vi "TalonSRXSetStatusRates.vi"(9 "Talon SRX Set Status Rates":T1={"General (ms)"=10, "Feedback 0 (ms)"=5, "Ain, Temp, Vbat (ms)"=255, "Misc (ms)"=255, "Comm Status (ms)"=255, "Mot Prof Buffer (ms)"=255, "Motion Magic (ms)"=255, "Firmware API Status (ms)"=255, "PIDF 1 (ms)"=255, "PIDF 0 (ms)"=255, "Feedback 1 (ms)"=255}, 11 "Talon SRX DevRef In":T2={"DeviceStatus"={"status"=FALSE, "code"=0, "source"=""}, "Type"=enum."PWM", "PWM"={"PWM Channel"=enum."PWM 1", "DeadBand"={"Name"="", "maxPositivePwm"=0, "minPositivePwm"=0, "centerPwm"=0, "maxNegativePwm"=0, "minNegativePwm"=0, "angularRange"=0}}, "CAN"={"Device Number"=0, "SetOutput VI Ref"=variant(enum8{"Percent VBus", "Current", "Speed", "Position", "Voltage"} enum."Percent VBus"), "GetOutput VI Ref"=variant(refnum<k1> refnum), "Enable VI Ref"=variant(dbl 12.0), "Disable VI Ref"=variant(enum8{"Percent VBus", "Speed", "Position", "Slave", "Unchanged / Invalid", "Voltage Compensation", "Current", "Motion Profile"} enum."Percent VBus"), "Data"=variant}, "Invert"=FALSE, "DIO PWM"={"PWM \"Enable\" Channel"=enum."Invalid", "DIOChannel"=enum."Invalid", "PWM Rate"=0.0}}) -> (3 "Talon SRX DevRef Out":T2={"DeviceStatus"={"status"=FALSE, "code"=0, "source"=""}, "Type"=enum."PWM", "PWM"={"PWM Channel"=enum."PWM 1", "DeadBand"={"Name"="", "maxPositivePwm"=0, "minPositivePwm"=0, "centerPwm"=0, "maxNegativePwm"=0, "minNegativePwm"=0, "angularRange"=0}}, "CAN"={"Device Number"=0, "SetOutput VI Ref"=variant(enum8{"Percent VBus", "Current", "Speed", "Position", "Voltage"} enum."Percent VBus"), "GetOutput VI Ref"=variant(refnum<k1> refnum), "Enable VI Ref"=variant(dbl 12.0), "Disable VI Ref"=variant(enum8{"Percent VBus", "Speed", "Position", "Slave", "Unchanged / Invalid", "Voltage Compensation", "Current", "Motion Profile"} enum."Percent VBus"), "Data"=variant}, "Invert"=FALSE, "DIO PWM"={"PWM \"Enable\" Channel"=enum."Invalid", "DIOChannel"=enum."Invalid", "PWM Rate"=0.0}})   [LabVIEW 2018]
uses:
  <vilib>/Rock Robotics/WPI/MotorControl/WPI_MotorControlDeviceRef.ctl
  <vilib>/Rock Robotics/WPI/MotorControl/WPI_MotorControlType.ctl
  <vilib>/Rock Robotics/SystemInterfaces/DIO/FPGA_DIOPWMChannel.ctl
  <vilib>/Rock Robotics/WPI/PWM/WPI_PWMDeadband.ctl
  <vilib>/Rock Robotics/SystemInterfaces/DIO/FPGA_DIOChannel.ctl
  <vilib>/Rock Robotics/WPI/ThirdParty/Phoenix-LabVIEW/Motor Controller/Controls/CTRE_Phoenix_MotorControl_StatusFrame.ctl
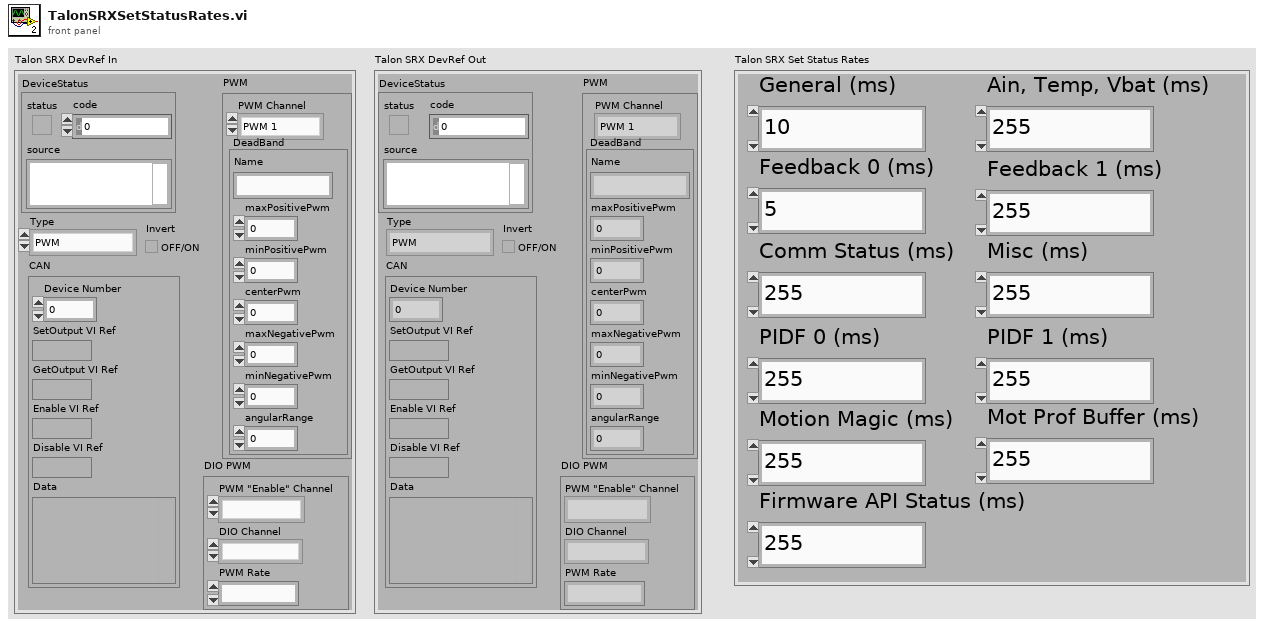
[diagram p1: front panel]
types:
  T1 = cluster{"General (ms)":i32, "Feedback 0 (ms)":i32, "Ain, Temp, Vbat (ms)":i32, "Misc (ms)":i32, "Comm Status (ms)":i32, "Mot Prof Buffer (ms)":i32, "Motion Magic (ms)":i32, "Firmware API Status (ms)":i32, "PIDF 1 (ms)":i32, "PIDF 0 (ms)":i32, "Feedback 1 (ms)":i32}
  T2 = typedef "WPI_MotorControlDeviceRef.ctl" = cluster{"DeviceStatus":errorcluster, "Type":T3, "PWM":cluster{"PWM Channel":T4, "DeadBand":T5}, "CAN":cluster{"Device Number":u8, "SetOutput VI Ref":variant, "GetOutput VI Ref":variant, "Enable VI Ref":variant, "Disable VI Ref":variant, "Data":variant}, "Invert":bool, "DIO PWM":cluster{"PWM \"Enable\" Channel":T4, "DIOChannel":T6, "PWM Rate":dbl}}
  T3 = typedef "WPI_MotorControlType.ctl" = enum16{"PWM", "CAN", "DIO PWM"}
  T4 = typedef "FPGA_DIOPWMChannel.ctl" = enum8{"PWM 0", "PWM 1", "PWM 2", "PWM 3", "PWM 4", "PWM 5", "PWM 6", "PWM 7", "PWM 8", "PWM 9", "PWM MXP 0", "PWM MXP 1", "PWM MXP 2", "PWM MXP 3", "PWM MXP 4", "PWM MXP 5", "PWM MXP 6", "PWM MXP 7", "PWM MXP 8", "PWM MXP 9", "Invalid"}
  T5 = typedef "WPI_PWMDeadband.ctl" = cluster{"Name":string, "maxPositivePwm":i32, "minPositivePwm":i32, "centerPwm":i32, "maxNegativePwm":i32, "minNegativePwm":i32, "angularRange":u16}
  T6 = typedef "FPGA_DIOChannel.ctl" = enum8{"DIO 0", "DIO 1", "DIO 2", "DIO 3", "DIO 4", "DIO 5", "DIO 6", "DIO 7", "DIO 8", "DIO 9", "DIO MXP 0", "DIO MXP 1", "DIO MXP 2", "DIO MXP 3", "DIO MXP 4", "DIO MXP 5", "DIO MXP 6", "DIO MXP 7", "DIO MXP 8", "DIO MXP 9", "DIO MXP 10", "DIO MXP 11", "DIO MXP 12", "DIO MXP 13", "DIO MXP 14", "DIO MXP 15", "SPI Port CS1", "SPI Port CS2", "SPI Port CS3", "SPI Port MISO", "SPI Port MOSI", "Invalid"}
  T7 = typedef "CTRE_Phoenix_MotorControl_StatusFrame.ctl" = u16
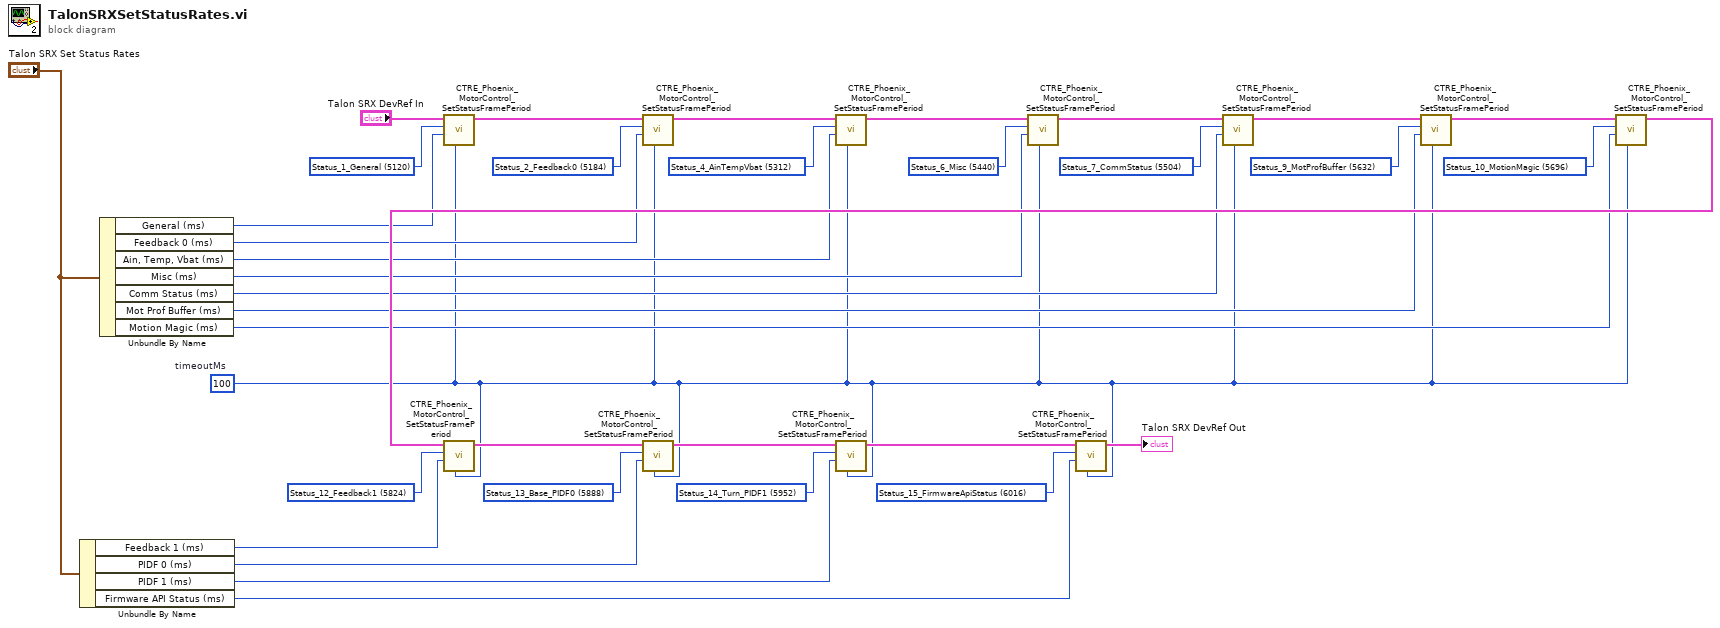
[diagram p0: block diagram]
diagram:
  w1 = 100  # timeoutMs
  w19 = T7 6016 items=["Status_1_General"=5120, "Status_2_Feedback0"=5184, "Status_4_AinTempVbat"=5312, "Status_6_Misc"=5440, "Status_7_CommStatus"=5504, "Status_9_MotProfBuffer"=5632, "Status_10_MotionMagic"=5696, "Status_12_Feedback1"=5824, "Status_13_Base_PIDF0"=5888, "Status_14_Turn_PIDF1"=5952, "Status_15_FirmwareApiStatus"=6016] ("Status Frame")
  w18 = T7 5952 items=["Status_1_General"=5120, "Status_2_Feedback0"=5184, "Status_4_AinTempVbat"=5312, "Status_6_Misc"=5440, "Status_7_CommStatus"=5504, "Status_9_MotProfBuffer"=5632, "Status_10_MotionMagic"=5696, "Status_12_Feedback1"=5824, "Status_13_Base_PIDF0"=5888, "Status_14_Turn_PIDF1"=5952, "Status_15_FirmwareApiStatus"=6016] ("Status Frame")
  w17 = T7 5888 items=["Status_1_General"=5120, "Status_2_Feedback0"=5184, "Status_4_AinTempVbat"=5312, "Status_6_Misc"=5440, "Status_7_CommStatus"=5504, "Status_9_MotProfBuffer"=5632, "Status_10_MotionMagic"=5696, "Status_12_Feedback1"=5824, "Status_13_Base_PIDF0"=5888, "Status_14_Turn_PIDF1"=5952, "Status_15_FirmwareApiStatus"=6016] ("Status Frame")
  w16 = T7 5824 items=["Status_1_General"=5120, "Status_2_Feedback0"=5184, "Status_4_AinTempVbat"=5312, "Status_6_Misc"=5440, "Status_7_CommStatus"=5504, "Status_9_MotProfBuffer"=5632, "Status_10_MotionMagic"=5696, "Status_12_Feedback1"=5824, "Status_13_Base_PIDF0"=5888, "Status_14_Turn_PIDF1"=5952, "Status_15_FirmwareApiStatus"=6016] ("Status Frame")
  w30 = T7 5696 items=["Status_1_General"=5120, "Status_2_Feedback0"=5184, "Status_4_AinTempVbat"=5312, "Status_6_Misc"=5440, "Status_7_CommStatus"=5504, "Status_9_MotProfBuffer"=5632, "Status_10_MotionMagic"=5696, "Status_12_Feedback1"=5824, "Status_13_Base_PIDF0"=5888, "Status_14_Turn_PIDF1"=5952, "Status_15_FirmwareApiStatus"=6016] ("Status Frame")
  w31 = T7 5632 items=["Status_1_General"=5120, "Status_2_Feedback0"=5184, "Status_4_AinTempVbat"=5312, "Status_6_Misc"=5440, "Status_7_CommStatus"=5504, "Status_9_MotProfBuffer"=5632, "Status_10_MotionMagic"=5696, "Status_12_Feedback1"=5824, "Status_13_Base_PIDF0"=5888, "Status_14_Turn_PIDF1"=5952, "Status_15_FirmwareApiStatus"=6016] ("Status Frame")
  w32 = T7 5504 items=["Status_1_General"=5120, "Status_2_Feedback0"=5184, "Status_4_AinTempVbat"=5312, "Status_6_Misc"=5440, "Status_7_CommStatus"=5504, "Status_9_MotProfBuffer"=5632, "Status_10_MotionMagic"=5696, "Status_12_Feedback1"=5824, "Status_13_Base_PIDF0"=5888, "Status_14_Turn_PIDF1"=5952, "Status_15_FirmwareApiStatus"=6016] ("Status Frame")
  w33 = T7 5440 items=["Status_1_General"=5120, "Status_2_Feedback0"=5184, "Status_4_AinTempVbat"=5312, "Status_6_Misc"=5440, "Status_7_CommStatus"=5504, "Status_9_MotProfBuffer"=5632, "Status_10_MotionMagic"=5696, "Status_12_Feedback1"=5824, "Status_13_Base_PIDF0"=5888, "Status_14_Turn_PIDF1"=5952, "Status_15_FirmwareApiStatus"=6016] ("Status Frame")
  w34 = T7 5312 items=["Status_1_General"=5120, "Status_2_Feedback0"=5184, "Status_4_AinTempVbat"=5312, "Status_6_Misc"=5440, "Status_7_CommStatus"=5504, "Status_9_MotProfBuffer"=5632, "Status_10_MotionMagic"=5696, "Status_12_Feedback1"=5824, "Status_13_Base_PIDF0"=5888, "Status_14_Turn_PIDF1"=5952, "Status_15_FirmwareApiStatus"=6016] ("Status Frame")
  w35 = T7 5184 items=["Status_1_General"=5120, "Status_2_Feedback0"=5184, "Status_4_AinTempVbat"=5312, "Status_6_Misc"=5440, "Status_7_CommStatus"=5504, "Status_9_MotProfBuffer"=5632, "Status_10_MotionMagic"=5696, "Status_12_Feedback1"=5824, "Status_13_Base_PIDF0"=5888, "Status_14_Turn_PIDF1"=5952, "Status_15_FirmwareApiStatus"=6016] ("Status Frame")
  w36 = T7 5120 items=["Status_1_General"=5120, "Status_2_Feedback0"=5184, "Status_4_AinTempVbat"=5312, "Status_6_Misc"=5440, "Status_7_CommStatus"=5504, "Status_9_MotProfBuffer"=5632, "Status_10_MotionMagic"=5696, "Status_12_Feedback1"=5824, "Status_13_Base_PIDF0"=5888, "Status_14_Turn_PIDF1"=5952, "Status_15_FirmwareApiStatus"=6016] ("Status Frame")
  n1 = Unbundle By Name("Talon SRX Set Status Rates") -> ("Feedback 1 (ms)"=w6:i32, "PIDF 0 (ms)"=w5:i32, "PIDF 1 (ms)"=w4:i32, "Firmware API Status (ms)"=w3:i32)
  n2 = Unbundle By Name("Talon SRX Set Status Rates") -> ("General (ms)"=w13:i32, "Feedback 0 (ms)"=w12:i32, "Ain, Temp, Vbat (ms)"=w11:i32, "Misc (ms)"=w10:i32, "Comm Status (ms)"=w9:i32, "Mot Prof Buffer (ms)"=w8:i32, "Motion Magic (ms)"=w7:i32)
  n3 = call <vilib>:"CTRE_Phoenix_MotorControl_SetStatusFramePeriod.vi"("timeoutMs"=w1, "periodMs"=w13, "Status Frame"=w36, "PhoenixMotorControlDevRef"="Talon SRX DevRef In") -> ("PhoenixMotorControlDevRef"=w24:T2)  [unwired: 6 in, 1 out]
  n4 = call <vilib>:"CTRE_Phoenix_MotorControl_SetStatusFramePeriod.vi"("timeoutMs"=w1, "periodMs"=w12, "Status Frame"=w35, "PhoenixMotorControlDevRef"=w24) -> ("PhoenixMotorControlDevRef"=w25:T2)  [unwired: 6 in, 1 out]
  n5 = call <vilib>:"CTRE_Phoenix_MotorControl_SetStatusFramePeriod.vi"("timeoutMs"=w1, "periodMs"=w11, "Status Frame"=w34, "PhoenixMotorControlDevRef"=w25) -> ("PhoenixMotorControlDevRef"=w26:T2)  [unwired: 6 in, 1 out]
  n6 = call <vilib>:"CTRE_Phoenix_MotorControl_SetStatusFramePeriod.vi"("timeoutMs"=w1, "periodMs"=w10, "Status Frame"=w33, "PhoenixMotorControlDevRef"=w26) -> ("PhoenixMotorControlDevRef"=w27:T2)  [unwired: 6 in, 1 out]
  n7 = call <vilib>:"CTRE_Phoenix_MotorControl_SetStatusFramePeriod.vi"("timeoutMs"=w1, "periodMs"=w9, "Status Frame"=w32, "PhoenixMotorControlDevRef"=w27) -> ("PhoenixMotorControlDevRef"=w28:T2)  [unwired: 6 in, 1 out]
  n8 = call <vilib>:"CTRE_Phoenix_MotorControl_SetStatusFramePeriod.vi"("timeoutMs"=w1, "periodMs"=w8, "Status Frame"=w31, "PhoenixMotorControlDevRef"=w28) -> ("PhoenixMotorControlDevRef"=w29:T2)  [unwired: 6 in, 1 out]
  n9 = call <vilib>:"CTRE_Phoenix_MotorControl_SetStatusFramePeriod.vi"("timeoutMs"=w1, "periodMs"=w7, "Status Frame"=w30, "PhoenixMotorControlDevRef"=w29) -> ("PhoenixMotorControlDevRef"=w14:T2)  [unwired: 6 in, 1 out]
  n10 = call <vilib>:"CTRE_Phoenix_MotorControl_SetStatusFramePeriod.vi"("timeoutMs"=w1, "periodMs"=w6, "Status Frame"=w16, "PhoenixMotorControlDevRef"=w14) -> ("PhoenixMotorControlDevRef"=w22:T2)  [unwired: 6 in, 1 out]
  n11 = call <vilib>:"CTRE_Phoenix_MotorControl_SetStatusFramePeriod.vi"("timeoutMs"=w1, "periodMs"=w5, "Status Frame"=w17, "PhoenixMotorControlDevRef"=w22) -> ("PhoenixMotorControlDevRef"=w21:T2)  [unwired: 6 in, 1 out]
  n12 = call <vilib>:"CTRE_Phoenix_MotorControl_SetStatusFramePeriod.vi"("timeoutMs"=w1, "periodMs"=w4, "Status Frame"=w18, "PhoenixMotorControlDevRef"=w21) -> ("PhoenixMotorControlDevRef"=w20:T2)  [unwired: 6 in, 1 out]
  n13 = call <vilib>:"CTRE_Phoenix_MotorControl_SetStatusFramePeriod.vi"("timeoutMs"=w1, "periodMs"=w3, "Status Frame"=w19, "PhoenixMotorControlDevRef"=w20) -> ("PhoenixMotorControlDevRef"=→"Talon SRX DevRef Out":T2)  [unwired: 6 in, 1 out]
